vi "Trigger logic - counter.vi"(8 "mode.continuous":bool, 9 "stream.enable":bool=TRUE, 10 "trig.samples.to.acq":u64, 11 "trig.sw start trigger":bool) -> (3 "enable out":bool)   [LabVIEW 2015, in "DDC_7976R_v1.lvlib"]
doc: "If \"Contonuous\" is true then \"Enable out\" always true,\nelse the counter defines the output."
uses:
  DDC_7976R_v1.lvlib
  <instrlib>/_niInstr/Basic Elements/v1/FPGA/Private/Count Down U64.vi
  <instrlib>/_niInstr/Basic Elements/v1/FPGA/niInstr Basic Elements v1 FPGA.lvlib
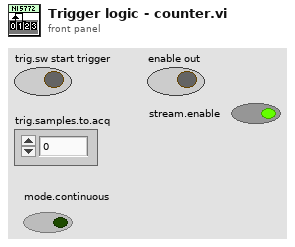
[diagram p1: front panel]
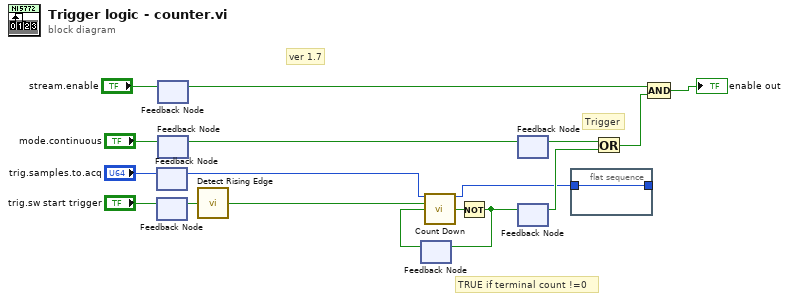
[diagram p0: block diagram]
diagram:
  # "ver 1.7"
  # "TRUE if terminal count !=0"
  # "Trigger"
  n1 = feedback #1() -> (w9:u64)  [unwired: 1 in]
  n2 = feedback-in #1("trig.samples.to.acq") -> ()
  n3 = feedback #2() -> (w10:bool)  [unwired: 1 in]
  n4 = feedback-in #2("trig.sw start trigger") -> ()
  n5 = feedback #3() -> (w1:bool)  [unwired: 1 in]
  n6 = feedback-in #3("stream.enable") -> ()
  n7 = feedback #4() -> (w12:bool)  [unwired: 1 in]
  n8 = feedback-in #4("mode.continuous") -> ()
  n9 = call <instrlib>:"Detect Rising Edge.vi"("signal"=w10) -> ("edge detected"=w8:bool)  [unwired: 14 in]
  n10 = feedback #5() -> (w6:bool)  [unwired: 1 in]
  n11 = call-poly <instrlib>:"Count Down.vi"("count in"=w9, "load"=w8, "decrement"=w6) -> ("count out"=w7:u64, "terminal count"=w14:bool)  [unwired: 11 in]
  n12 = Not(x=w14) -> (.not. x?=w5:bool)
  n13 = feedback-in #5(w5) -> ()
  n14 = feedback #6() -> (w16:bool)  [unwired: 1 in]
  n15 = feedback-in #6(w12) -> ()
  n16 = feedback #7() -> (w15:bool)  [unwired: 1 in]
  n17 = feedback-in #7(w5) -> ()
  n18 = flat-sequence {
    tunnel: w7 -> [w18]
    tunnel: [w18] -> _
    frame #0 {
    }
  }
  n19 = Or(x=w16, y=w15) -> (x .or. y?=w3:bool)
  n20 = Compound Arithmetic op=AND(w1, w3) -> (→"enable out":bool)
